vi "UpdateTECsp.vi"(7 "LVWS Req":refnum<class "Web Request.lvclass">, 11 "TECsp":string) -> ()   [LabVIEW 2014]
uses:
  Controller/Controller.lvclass
  Controller/Controls/Enqueuer Enum.ctl
  <vilib>/wsapi/Web Request.lvclass
  Instr Actor/Messages/Set TEC SP MSG2/Set TEC SP MSG.lvclass
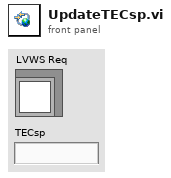
[diagram p1: front panel]
types:
  T1 = typedef "Controller.lvlib/Controller.lvclass/Enqueuer Enum.ctl" = enum8{"PAS", "CRDS", "File", "O3Lamp"}
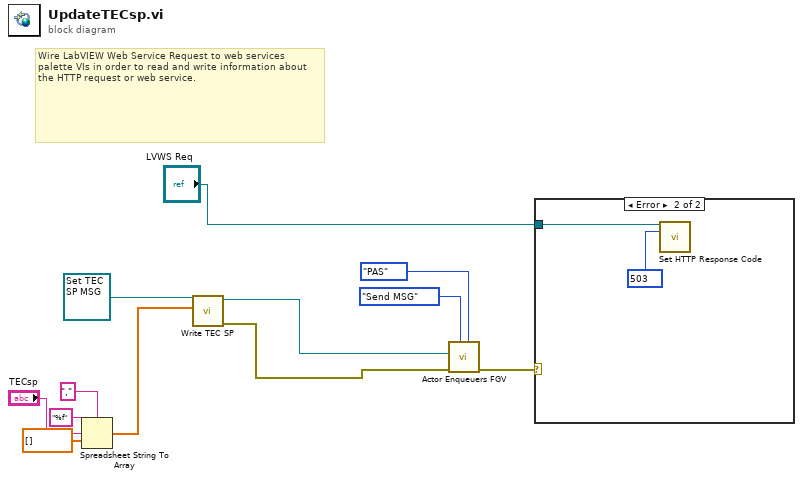
[diagram p0: block diagram]
diagram:
  # "Wire LabVIEW Web Service Request to web services palette VIs in order to read and write information about the HTTP request or web service."
  n1 = Spreadsheet String To Array(delimiter (Tab)=",", format string="%f", spreadsheet string="TECsp", array type (2D Dbl)=dbl[] []) -> (array=w3:dbl[])
  n2 = call "Write TEC SP.vi"("TEC SP"=w3, "Set TEC SP MSG in"=refnum<class "Set TEC SP MSG.lvclass"> refnum ("Instrument Lib:Set TEC SP MSG.lvclass")) -> ("error out"=w1:errorcluster, "Set TEC SP MSG out"=w2:refnum<class "Set TEC SP MSG.lvclass">)  [unwired: 8 in]
  n3 = call "Actor Enqueuers FGV.vi"("Enqueuer"=Enqueuer_Enum."PAS", "State"=enum16{"Store", "Send MSG"}."Send MSG", "error in"=w1, "MSG"=w2) -> ("error out"=w10:errorcluster)  [unwired: 7 in]
  n4 = case shown="Error" w10 {
    tunnel: "LVWS Req" -> [_ w13]
    frame No Error {
    }
    frame Error {
      w14 = 503 items=["100"=100, "101"=101, "200"=200, "201"=201, "202"=202, "203"=203, "204"=204, "205"=205, "206"=206, "300"=300, "301"=301, "302"=302, "303"=303, "304"=304, "305"=305, "306"=306, "307"=307, "400"=400, "401"=401, "402"=402, "403"=403, "404"=404, "405"=405, "406"=406, "407"=407, "408"=408, "409"=409, "410"=410, "411"=411, "412"=412, "413"=413, "414"=414, "415"=415, "416"=416, "417"=417, "500"=500, "501"=501, "502"=502, "503"=503, "504"=504, "505"=505] ("response code (200)")
      n5 = call <vilib>:"Set HTTP Response Code.vi"("LabVIEW Web Service Request"=w13, "response code (200)"=w14) -> ()  [unwired: 12 in, 2 out]
    }
  }
